vi "YellowState_Init.vi"(0 "object in":refnum<class "YellowState.lvclass">, 2 "TrafficLight":refnum<class "TrafficLight.lvclass">, 5 "Error In":errorcluster) -> (14 "object out":refnum<class "YellowState.lvclass">, 19 "Error Out":errorcluster)   [LabVIEW 2024, in "YellowState.lvclass"]
uses:
  YellowState.lvclass
  C:/Users/burakkorkmaz/Desktop/Leveling/labview-desing-patterns/State Pattern/State_interface/State.lvclass
  TrafficLight_class/TrafficLight.lvclass
  YellowState.lvclass/YellowState.ctl
panel:
  # "Connector Pane"
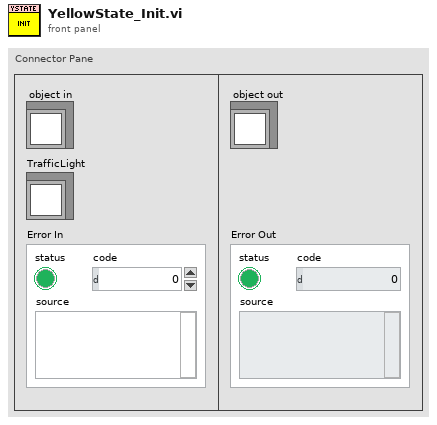
[diagram p1: front panel]
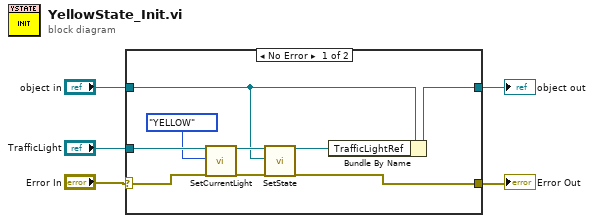
[diagram p0: block diagram]
diagram:
  n1 = case shown="No Error" "Error In" {
    selector: "Error In" -> [w13 w15]
    tunnel: "object in" -> [w7 w16]
    tunnel: [w14 w16] -> w4
    tunnel: [w10 w15] -> w2
    tunnel: "TrafficLight" -> [w11 _]
    frame No Error {
      n2 = call-dynamic "SetCurrentLight.vi"("object in"=w11, "CurrentLight"=enum16{"RED", "YELLOW", "GREEN"}."YELLOW", "Error In"=w13) -> ("object out"=w9:refnum<class "TrafficLight.lvclass">, "Error Out"=w12:errorcluster)  [unwired: 15 in]
      n3 = call-dynamic "SetState.vi"("object in"=w9, "State"=w7, "Error In"=w12) -> ("object out"=w8:refnum<class "TrafficLight.lvclass">, "Error Out"=w10:errorcluster)  [unwired: 15 in]
      n4 = Bundle By Name(cluster=w7, "TrafficLightRef"=w8) -> (w14:refnum<class "YellowState.lvclass">)
    }
    frame Error {
    }
  }
  "object out" <- w4
  "Error Out" <- w2
